vi "Drawbridge Controller Initialization.vi"(10 "Subsystem Name":string, 11 "Default Command":T1) -> (3 "Command Info":T6)   [LabVIEW 2015]
uses:
  Drawbridge Setpoints.ctl
  Drawbridge Operations.ctl
  <vilib>/Rock Robotics/WPI/Framework/Command Status Info.ctl
  <vilib>/Rock Robotics/WPI/Framework/Completion Status.ctl
  <vilib>/Rock Robotics/WPI/Framework/Completion Notifier.ctl
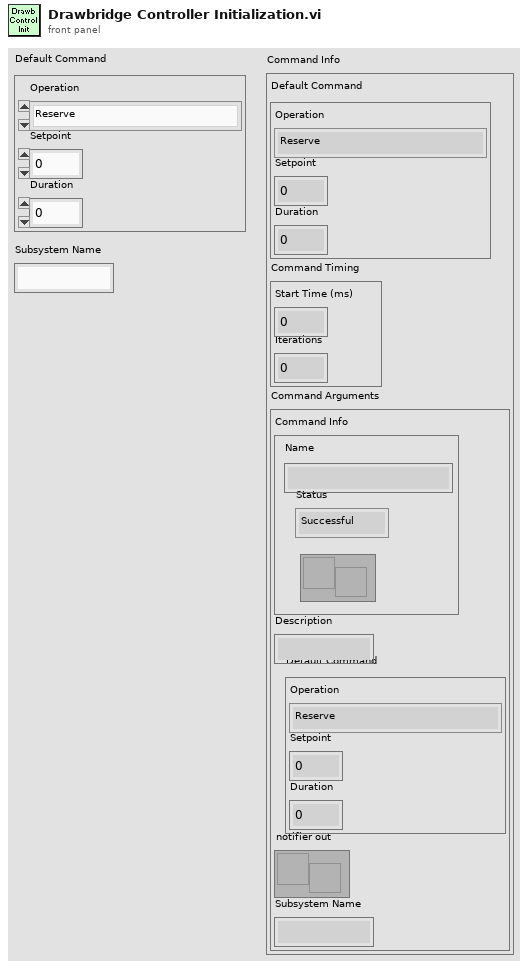
[diagram p1: front panel]
types:
  T1 = typedef "Drawbridge Setpoints.ctl" = cluster{"Operation":T2, "Setpoint":dbl, "Duration":dbl}
  T2 = typedef "Drawbridge Operations.ctl" = enum16{"Reserve", "Read Current", "Immediate", "Open"}
  T3 = typedef "Command Status Info.ctl" = cluster{"Name":string, "Status":T4, "notifier out":T5}
  T4 = typedef "Completion Status.ctl" = enum16{"Successful", "Aborted", "Incomplete"}
  T5 = typedef "Completion Notifier.ctl" = refnum<notifier>
  T6 = cluster{"Default Command":T1, "Command Timing":cluster{"Start Time (ms)":u32, "Iterations":i32}, "Command Arguments":cluster{"Command Info":T3, "Description":string, "Default Command":T1, "notifier out":refnum<notifier>, "Subsystem Name":string}}
  T7 = cluster{"Default Command":T1, "Command Info":T3, "Description":string}
  T8 = cluster{"Command Info":T3, "Description":string, "Default Command":T1, "notifier out":refnum<notifier>, "Subsystem Name":string}
  T9 = cluster{"Default Command":T1, cluster{"Start Time (ms)":u32, "Iterations":i32}, cluster{"Command Info":T3, "Description":string, "Default Command":T1, "notifier out":refnum<notifier>, "Subsystem Name":string}}
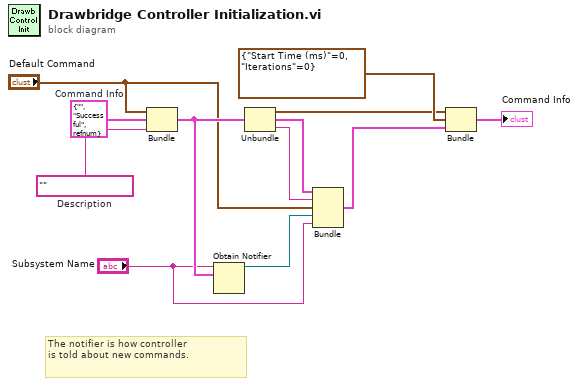
[diagram p0: block diagram]
diagram:
  w8 = T3 {"Name"="", "Status"=enum."Successful", "notifier out"=refnum}  # Command Info
  w9 = ""  # Description
  # "The notifier is how controller\nis told about new commands."
  n1 = Bundle("Default Command"="Default Command", "Command Info"=w8, "Description"=w9) -> (w10:T7)  [unwired: 1 in]
  n2 = Obtain Notifier(name (unnamed)="Subsystem Name", notification data type=w10) -> (notifier out=w3:refnum<notifier>)  [unwired: 2 in, 2 out]
  n3 = Unbundle(w10) -> ("Default Command"=w11:T1, "Command Info"=w4:T3, "Description"=w5:string)
  n4 = Bundle("Command Info"=w4, "Description"=w5, "Default Command"="Default Command", "notifier out"=w3, "Subsystem Name"="Subsystem Name") -> (w6:T8)  [unwired: 1 in]
  n5 = Bundle("Default Command"=w11, cluster{"Start Time (ms)":u32, "Iterations":i32} {"Start Time (ms)"=0, "Iterations"=0}, w6) -> (→"Command Info":T9)  [unwired: 1 in]
